vi "Close.vi"(8 "error in":errorcluster) -> (0 "error out":errorcluster)   [LabVIEW 2020, in "reporting-device.lvlib" / "VI Reference Management.lvlib"]
doc: "Close the master reference of the cloneable Main VI.\n_____\nBased on DQMH Project Template 7.0.1.1316."
uses:
  VI Reference Management.lvlib
  Action--enum.ctl
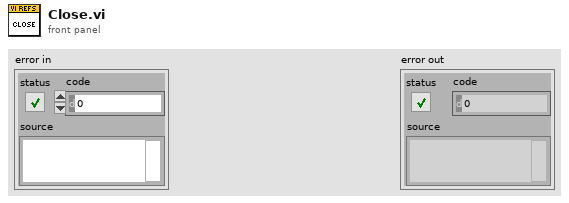
[diagram p1: front panel]
types:
  T1 = typedef "reporting-device.lvlib/VI Reference Management.lvlib/Action--enum.ctl" = enum16{"Get", "Create", "Close"}
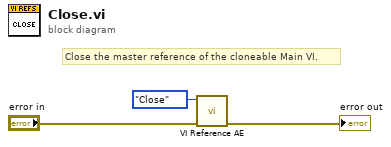
[diagram p0: block diagram]
diagram:
  # "Close the master reference of the cloneable Main VI."
  n1 = call "VI Reference AE.vi"("error in"="error in", "Action"=Action--enum."Close") -> ("error out"=→"error out":errorcluster)  [unwired: 7 in, 1 out]
